vi "AutofocusOptions.vi"() -> ()   [LabVIEW 2021, in "Test VIs.lvclass"]
uses:
  Test VIs/Test VIs.lvclass
  Drivers/Aerotech A3200/Aerotech.lvlib
  <vilib>/Utility/file.llb/Read Delimited Spreadsheet (DBL).vi
  <vilib>/vision/driver/NI_Vision_Acquisition_Software.lvlib
  <vilib>/userdefined/High Color/IMAQdx.ctl
panel:
  in  "Camera":T1="cam1"
  in  "DistSensorInTextFileMode":bool
  out "XYZ_NiterOrDistSenErr":string
  in  "AbortAutoFocus":bool
  in  "Tolerance":dbl=0.005 format="%#_13g"
  out "TimeTaken":dbl
  out "Z":string
  in  "SafeMaxZ":dbl=75.0 format="%#_13g"
  out "N_iterations":dbl[](array[numeric])
  in  "InitialStepSize":dbl=0.1
  out "HighVSPosition":picture
  in  "Z OutputFile":path=path "C:/Users/TTUHEP/Documents/LabVIEW/GantryPrograms/LogFiles/temp.txt"
  in  "PlotOutputFile":string="C:\\Users\\TTUHEP\\Documents\\LabVIEW\\GantryPrograms\\LogFiles\\plot.png"
  in  "Zoffset_textFile":dbl
  out "Image":T2(plugin-control)
  in  "InitialPositions":path=path "C:/Users/TTUHEP/Documents/LabVIEW/GantryPrograms/Configs/A1_BP_HeightMeasure.txt"
  out "error out":errorcluster
  out "BestZvalue":dbl
  in  "error in (no error)":errorcluster
  in  "Z":dbl=68.683
  in  "Y":dbl=1011.604463
  in  "X":dbl=288.7508563
  in  "ControlType":T3(ring)=enum."SinglePoint" caption="Operation Mode"
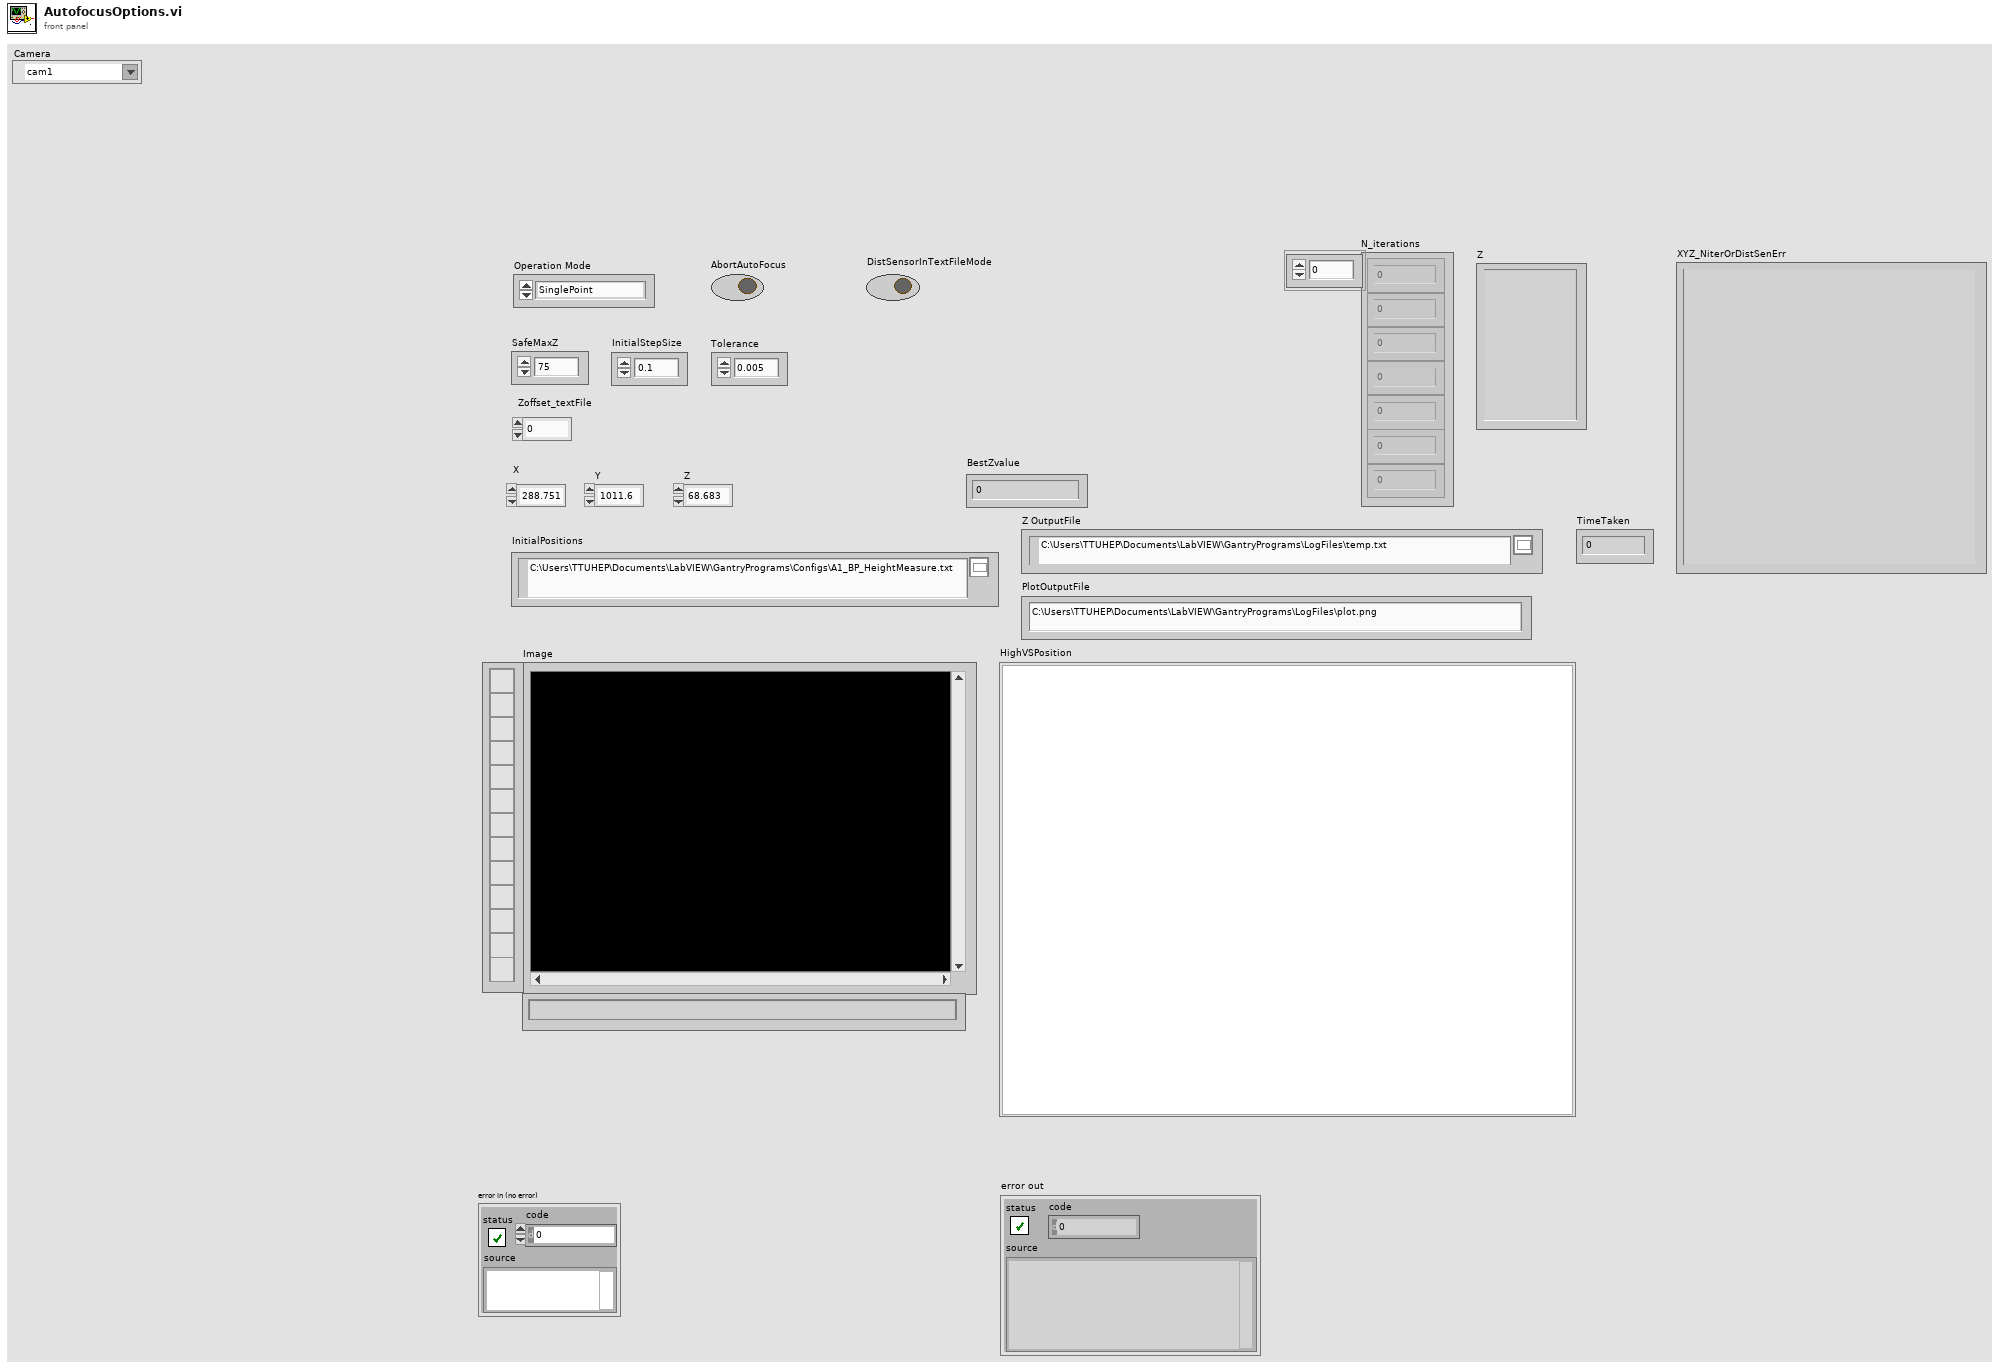
[diagram p1: front panel]
types:
  T1 = typedef "IMAQdx.ctl" = refnum<k21>
  T2 = typedef "IMAQ Image.ctl" = refnum<image>
  T3 = enum16{"CurrentPosition", "SinglePoint", "TextFile"}
  T4 = typedef "Image Type" = u32
  T5 = enum16{"open", "replace", "create", "open or create", "replace or create", "replace or create with confirmation"}
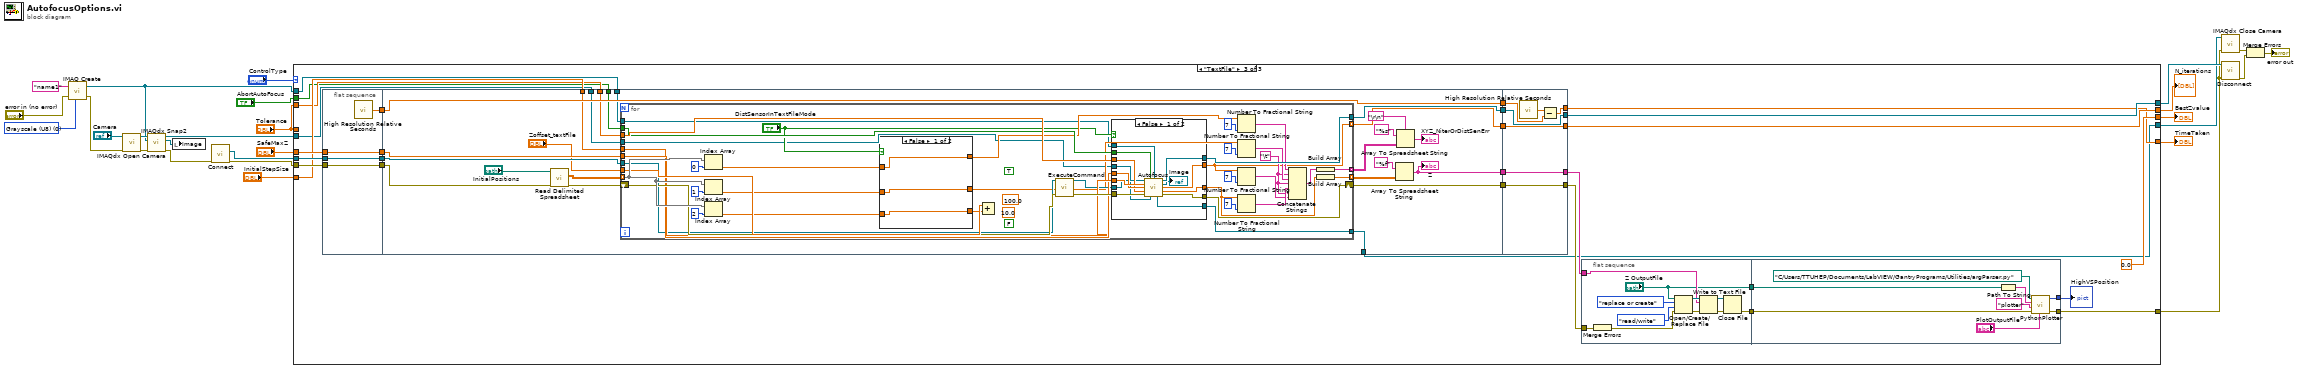
[diagram p0: block diagram]
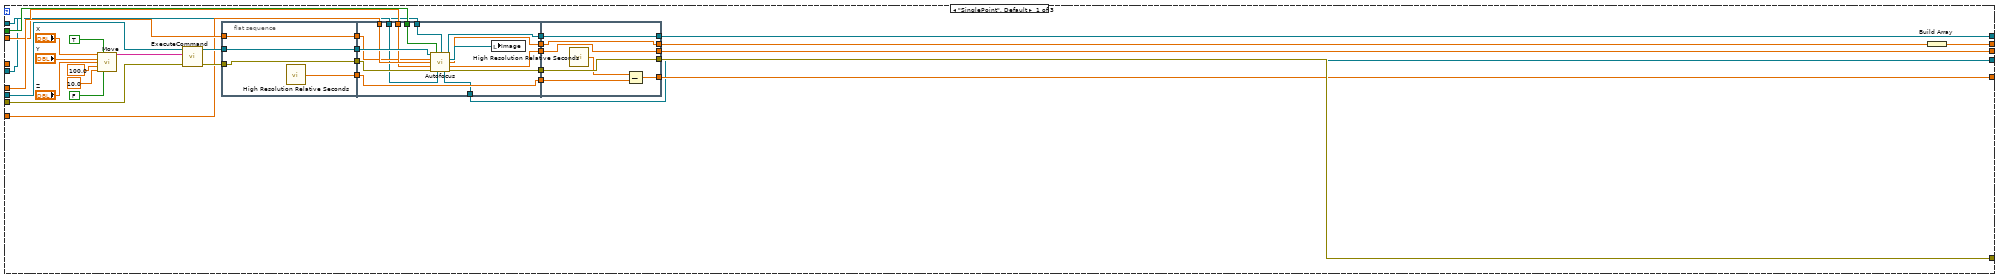
[diagram p2: hidden frame]
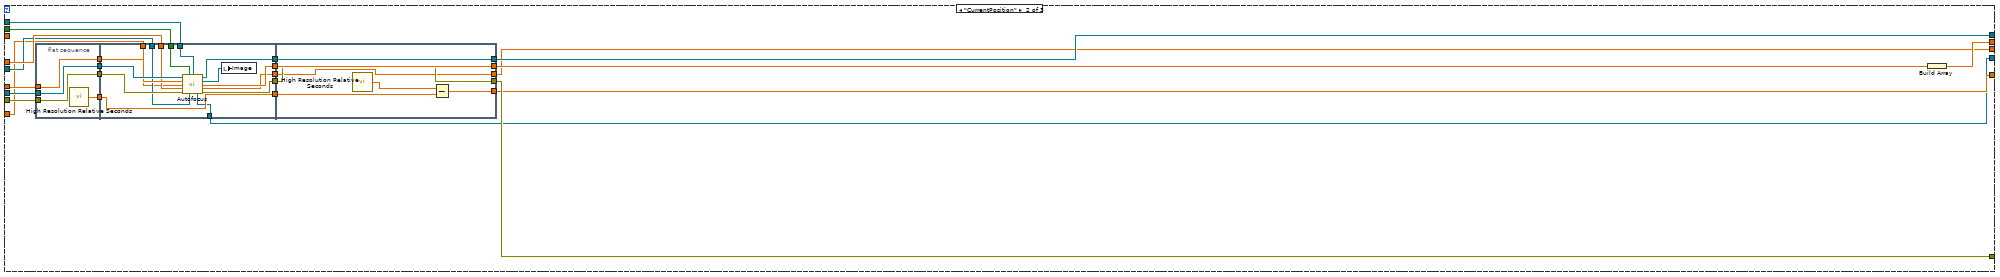
[diagram p3: hidden frame]
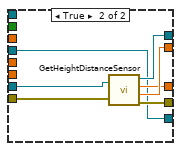
[diagram p4: hidden frame]
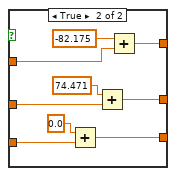
[diagram p5: hidden frame]
diagram:
  w13 = T4 0 items=["Grayscale (U8)", "Grayscale (I16)", "Grayscale (SGL)", "Complex (CSG)", "RGB (U32)", "HSL (U32)", "RGB (U64)", "Grayscale (U16)"] ("Image Type")
  n1 = call "IMAQ Create"("Image Name"="name1" ("ImageName"), "Image Type"=w13, "error in (no error)"="error in (no error)") -> ("New Image"=w5:T2, "error out"=w15:errorcluster)  [unwired: 2 in]
  n2 = call <vilib>:"IMAQdx Open Camera.vi"("error in"=w15, "Session In"="Camera") -> ("error out"=w4:errorcluster, "Session Out"=w6:T1)  [unwired: 8 in]
  n3 = call <vilib>:"IMAQdx Snap2.vi"("error in"=w4, "Image In"=w5, "Session In"=w6) -> ("error out"=w3:errorcluster, "Image Out"=w1:T2, "Session Out"=w2:T1)  [unwired: 6 in]
  n4 = local write "Image"(w1) -> ()
  n5 = call "Connect.vi"("error in (no error)"=w3) -> ("error out"=w25:errorcluster, "controller"=w26:refnum<k24>)  [unwired: 9 in]
  n6 = case shown="\"TextFile\"" "ControlType" {
    tunnel: w25 -> [w35 w109 w160]
    tunnel: [w61 w105 w156] -> w9
    tunnel: w26 -> [w45 w110 w164]
    tunnel: [w60 w106 w163] -> w24
    tunnel: [w58 w107 w161] -> w23
    tunnel: "SafeMaxZ" -> [w57 w108 w159]
    tunnel: [w56 w104 0.0 ("BestZvalue")] -> w21
    tunnel: [w46 w94 w144] -> w20
    tunnel: "Tolerance" -> [_ w93 _]
    tunnel: "InitialStepSize" -> [w33 w88 w143]
    tunnel: "Tolerance" -> [w32 _ w142]
    tunnel: "AbortAutoFocus" -> [w31 w92 w141]
    tunnel: w2 -> [w30 w91 w140]
    tunnel: w5 -> [w29 w90 w139]
    tunnel: [w28 w89 w138] -> w11
    frame "SinglePoint", Default {
      n7 = call "Move.vi"("X"="X", "Absolute"=TRUE, "Y"="Y", "Z"="Z", "SpeedXY (mm/s)"=100.0, "SpeedZ (mm/s)"=10.0, "Move Z first"=FALSE) -> ("Position Gcode"=w36:string)  [unwired: 8 in]
      n8 = call "ExecuteCommand.vi"("error in (no error)"=w35, "Command Code"=w36, "controller in"=w45) -> ("error out"=w34:errorcluster, "controller out"=w44:refnum<k24>)  [unwired: 6 in, 1 out]
      n9 = flat-sequence {
        tunnel: w57 -> [w64]
        tunnel: w44 -> [w65]
        tunnel: [w62] -> w55
        tunnel: [w65] -> w54
        tunnel: [w64] -> w53
        tunnel: [w63] -> w47
        tunnel: w34 -> [w62]
        tunnel: w55 -> [w80]
        tunnel: w54 -> [w73]
        tunnel: w53 -> [w70]
        tunnel: [w79] -> w52
        tunnel: [w78] -> w51
        tunnel: [w76] -> w50
        tunnel: [w75] -> w49
        tunnel: [w74] -> w48
        tunnel: w47 -> [w74]
        tunnel: w33 -> [w72]
        tunnel: w32 -> [w71]
        tunnel: w31 -> [w69]
        tunnel: w30 -> [w68]
        tunnel: w29 -> [w67]
        tunnel: [w66] -> w28
        tunnel: [w84] -> w56
        tunnel: [w85] -> w59
        tunnel: [w86] -> w60
        tunnel: [w87] -> w61
        tunnel: w52 -> [w87]
        tunnel: w51 -> [w86]
        tunnel: w50 -> [w85]
        tunnel: w49 -> [w84]
        tunnel: w48 -> [w82]
        tunnel: [w81] -> w46
        frame #0 {
          n10 = call <vilib>:"High Resolution Relative Seconds.vi"() -> ("relative seconds"=w63:dbl)
        }
        frame #1 {
          n11 = call "Autofocus.vi"("controller in"=w73, "AbortAutoFocus"=w69, "ImageIn"=w67, "SafeMaxZ"=w70, "InitialStepSize"=w72, "Tolerance"=w71, "error in (no error)"=w80, "SessionIn"=w68) -> ("controller out"=w78:refnum<k24>, "Image"=w77:T2, "N_iterations"=w76:dbl, "BestZvalue"=w75:dbl, "Session Out"=w66:T1, "error out"=w79:errorcluster)  [unwired: 2 in]
          n12 = local write "Image"(w77) -> ()
        }
        frame #2 {
          n13 = call <vilib>:"High Resolution Relative Seconds.vi"() -> ("relative seconds"=w83:dbl)
          n14 = Subtract(x=w83, y=w82) -> (x-y=w81:dbl)
        }
      }
      n15 = Build Array(w59) -> (w58:dbl[])
    }
    frame "CurrentPosition" {
      n16 = flat-sequence {
        tunnel: w108 -> [w113]
        tunnel: w109 -> [w114]
        tunnel: w110 -> [w115]
        tunnel: [w115] -> w103
        tunnel: [w114] -> w102
        tunnel: [w113] -> w101
        tunnel: [w112] -> w96
        tunnel: w103 -> [w124]
        tunnel: w102 -> [w123]
        tunnel: w101 -> [w122]
        tunnel: [w129] -> w100
        tunnel: [w128] -> w99
        tunnel: [w127] -> w98
        tunnel: [w126] -> w97
        tunnel: w96 -> [w125]
        tunnel: [w125] -> w95
        tunnel: w93 -> [w121]
        tunnel: w92 -> [w120]
        tunnel: w91 -> [w119]
        tunnel: w90 -> [w118]
        tunnel: [w117] -> w89
        tunnel: w88 -> [w116]
        tunnel: [w134] -> w104
        tunnel: [w135] -> w105
        tunnel: [w136] -> w106
        tunnel: [w137] -> w111
        tunnel: w100 -> [w137]
        tunnel: w99 -> [w136]
        tunnel: w98 -> [w135]
        tunnel: w97 -> [w134]
        tunnel: w95 -> [w132]
        tunnel: [w131] -> w94
        frame #0 {
          n17 = call <vilib>:"High Resolution Relative Seconds.vi"() -> ("relative seconds"=w112:dbl)
        }
        frame #1 {
          n18 = call "Autofocus.vi"("controller in"=w124, "AbortAutoFocus"=w120, "ImageIn"=w118, "SafeMaxZ"=w122, "InitialStepSize"=w116, "Tolerance"=w121, "error in (no error)"=w123, "SessionIn"=w119) -> ("controller out"=w128:refnum<k24>, "Image"=w130:T2, "N_iterations"=w129:dbl, "BestZvalue"=w126:dbl, "Session Out"=w117:T1, "error out"=w127:errorcluster)  [unwired: 2 in]
          n19 = local write "Image"(w130) -> ()
        }
        frame #2 {
          n20 = call <vilib>:"High Resolution Relative Seconds.vi"() -> ("relative seconds"=w133:dbl)
          n21 = Subtract(x=w133, y=w132) -> (x-y=w131:dbl)
        }
      }
      n22 = Build Array(w111) -> (w107:dbl[])
    }
    frame "TextFile" {
      n23 = flat-sequence {
        tunnel: w159 -> [w167]
        tunnel: w160 -> [w168]
        tunnel: w164 -> [w169]
        tunnel: [w169] -> w153
        tunnel: [w168] -> w152
        tunnel: [w167] -> w151
        tunnel: [w166] -> w146
        tunnel: w153 -> [w191]
        tunnel: w152 -> [w187]
        tunnel: w151 -> [w185]
        tunnel: [w173] -> w150
        tunnel: [w190] -> w149
        tunnel: [w174] -> w148
        tunnel: [w188] -> w147
        tunnel: w146 -> [w182]
        tunnel: [w182] -> w145
        tunnel: w143 -> [w181]
        tunnel: w142 -> [w180]
        tunnel: w141 -> [w179]
        tunnel: w140 -> [w172]
        tunnel: w139 -> [w171]
        tunnel: [w170] -> w138
        tunnel: [w269] -> w161
        tunnel: [w270] -> w162
        tunnel: [w271] -> w163
        tunnel: [w272] -> w165
        tunnel: w150 -> [w272]
        tunnel: w149 -> [w271]
        tunnel: w148 -> [w270]
        tunnel: w147 -> [w269]
        tunnel: w145 -> [w267]
        tunnel: [w266] -> w144
        frame #0 {
          n24 = call <vilib>:"High Resolution Relative Seconds.vi"() -> ("relative seconds"=w166:dbl)
        }
        frame #1 {
          n25 = call-poly <vilib>:"Read Delimited Spreadsheet.vi"("file path (dialog if empty)"="InitialPositions", "error in (no error)"=w187) -> ("all rows"=w193:dbl[][], "error out"=w186:errorcluster)  [unwired: 8 in, 4 out]
          n26 = for {
            tunnel: w193 -> [w229] mode=indexing
            tunnel: [w228] -> w183 mode=indexing
            tunnel: w191 -> [w220]
            tunnel: [w227] -> w190
            tunnel: [w199] -> w188 mode=indexing
            tunnel: w185 -> [w223]
            tunnel: "Zoffset_textFile" -> [w226]
            tunnel: w181 -> [w222]
            tunnel: w180 -> [w221]
            tunnel: w179 -> [w218]
            tunnel: [w209] -> w178 mode=indexing
            shift-right: [w208] -> w173
            shift-left: w186 -> [w225]
            tunnel: w172 -> [w196]
            tunnel: w171 -> [w195]
            tunnel: [w194] -> w170
            w200 = "\t"
            (unwired) FALSE ("Move Z first")
            (unwired) TRUE ("Absolute")
            (unwired) 10.0 ("SpeedZ (mm/s)")
            (unwired) 100.0 ("SpeedXY (mm/s)")
            n27 = Index Array(array=w229, index=0) -> (element=w206:dbl)
            n28 = Index Array(array=w229, index=1) -> (element=w204:dbl)
            n29 = Index Array(array=w229, index=2) -> (element=w203:dbl)
            n30 = case shown="False" "DistSensorInTextFileMode" {
              tunnel: [w256 w264] -> w207
              tunnel: w206 -> [w256 w263]
              tunnel: [w255 w262] -> w205
              tunnel: w204 -> [w255 w260]
              tunnel: w203 -> [w254 w259]
              tunnel: [w254 w257] -> w202
              frame False {
              }
              frame True {
                n31 = Add(x=0.0, y=w259) -> (x+y=w257:dbl)
                n32 = Add(x=74.471, y=w260) -> (x+y=w262:dbl)
                n33 = Add(x=-82.175, y=w263) -> (x+y=w264:dbl)
              }
            }
            n34 = Add(x=w226, y=w202) -> ()  [unwired: 1 out]
            n35 = call "ExecuteCommand.vi"("error in (no error)"=w225, "controller in"=w220) -> ("error out"=w224:errorcluster, "controller out"=w219:refnum<k24>)  [unwired: 7 in, 1 out]
            n36 = case shown="False" "DistSensorInTextFileMode" {
              tunnel: [w246 w251] -> w227
              tunnel: [w245 w249] -> w199
              tunnel: w224 -> [w243 w252]
              tunnel: w223 -> [w242 _]
              tunnel: w222 -> [w241 _]
              tunnel: w221 -> [w240 _]
              tunnel: w219 -> [w239 w253]
              tunnel: w218 -> [w238 _]
              tunnel: [w237 w248] -> w215
              tunnel: [w236 w250] -> w208
              tunnel: w196 -> [w235 w247]
              tunnel: w195 -> [w234 _]
              tunnel: [w233 w247] -> w194
              frame False {
                n37 = call "Autofocus.vi"("controller in"=w239, "AbortAutoFocus"=w238, "ImageIn"=w234, "SafeMaxZ"=w242, "InitialStepSize"=w241, "Tolerance"=w240, "error in (no error)"=w243, "SessionIn"=w235) -> ("controller out"=w246:refnum<k24>, "Image"=→"Image":T2, "N_iterations"=w245:dbl, "BestZvalue"=w237:dbl, "Session Out"=w233:T1, "error out"=w236:errorcluster)  [unwired: 2 in]
              }
              frame True {
                n38 = call "GetHeightDistanceSensor.vi"("controller in"=w253, "error in (no error)"=w252) -> ("controller out"=w251:refnum<k24>, "MeanHeight(mm)"=w248:dbl, "SDofHeight(mm)"=w249:dbl, "error out"=w250:errorcluster)
              }
            }
            n39 = Number To Fractional String(number=w207, precision (6)=i16 7) -> (F-format string=w213:string)  [unwired: 2 in]
            n40 = Number To Fractional String(number=w205, precision (6)=i16 7) -> (F-format string=w212:string)  [unwired: 2 in]
            n41 = Number To Fractional String(number=w199, precision (6)=i16 7) -> (F-format string=w197:string)  [unwired: 2 in]
            n42 = Number To Fractional String(number=w215, precision (6)=i16 7) -> (F-format string=w211:string)  [unwired: 2 in]
            n43 = Concatenate Strings(w213, w200, w212, w200, w211, w200, w197) -> (w210:string)
            n44 = Build Array(w210) -> (w209:string[])
            n45 = Build Array(w215) -> (w228:dbl[])
          }
          n46 = Array To Spreadsheet String(array=w183, 3:"%f" ("format string")) -> (spreadsheet string=w174:string)  [unwired: 1 in]
          "Z" <- w174
          n47 = Array To Spreadsheet String(delimiter (Tab)="\r\n", array=w178, 3:"%s" ("format string")) -> (spreadsheet string=→"XYZ_NiterOrDistSenErr":string)
        }
        frame #2 {
          n48 = call <vilib>:"High Resolution Relative Seconds.vi"() -> ("relative seconds"=w268:dbl)
          n49 = Subtract(x=w268, y=w267) -> (x-y=w266:dbl)
        }
      }
      n50 = flat-sequence {
        tunnel: w165 -> [w283]
        tunnel: w162 -> [w276]
        tunnel: [w274] -> w157
        tunnel: ["Z OutputFile"] -> w154
        tunnel: w157 -> [w291]
        tunnel: [w290] -> w156
        tunnel: [w289] -> w155
        tunnel: w154 -> [w285]
        frame #0 {
          n51 = Merge Errors(w283) -> (w275:errorcluster)
          n52 = Open/Create/Replace File(file path (use dialog)="Z OutputFile", error in=w275, operation (0:open)=T5."replace or create", access (0:read/write)=enum16{"read/write", "read-only", "write-only"}."read/write") -> (refnum out=w279:refnum<file>, error out=w280:errorcluster)  [unwired: 2 in, 1 out]
          n53 = Write to Text File(file (use dialog)=w279, text=w276, error in=w280) -> (refnum out=w282:refnum<file>, error out=w281:errorcluster)  [unwired: 1 in, 1 out]
          n54 = Close File(refnum=w282, error in=w281) -> (error out=w274:errorcluster)  [unwired: 1 out]
        }
        frame #1 {
          n55 = Path To String(path=w285) -> (string=w286:string)
          n56 = call "PythonPlotter.vi"("Output File"="PlotOutputFile", "error in (no error)"=w291, "Function Name"="plotter", "Input File"=w286, "Python Path"=path "C:/Users/TTUHEP/Documents/LabVIEW/GantryPrograms/Utilities/argParser.py") -> ("error out"=w290:errorcluster, "HighVSPosition"=w289:picture)  [unwired: 4 in]
        }
      }
      "HighVSPosition" <- w155
    }
  }
  "N_iterations" <- w23
  "BestZvalue" <- w21
  "TimeTaken" <- w20
  n57 = call <vilib>:"IMAQdx Close Camera.vi"("error in"=w9, "Session In"=w11) -> ("error out"=w10:errorcluster)  [unwired: 9 in]
  n58 = call "Disconnect.vi"("error in (no error)"=w9, "controller"=w24) -> ("error out"=w8:errorcluster)  [unwired: 9 in]
  n59 = Merge Errors(w10, w8) -> (→"error out":errorcluster)
